vi "FIN UI.vi"() -> ()   [LabVIEW 2015]
panel:
  in  "Stop Button":bool
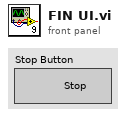
[diagram p1: front panel]
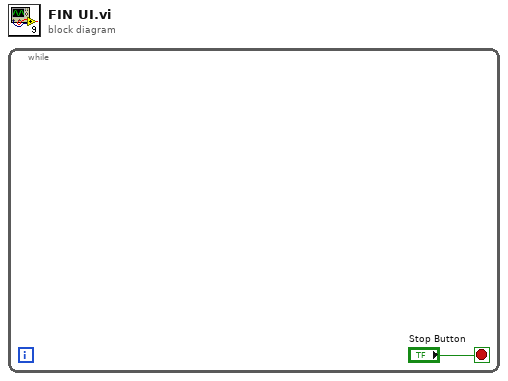
[diagram p0: block diagram]
diagram:
  n1 = while {
    stop <- "Stop Button" stop-if-true
  }
